vi "GetPositionWinCoords.vi"(8 "error in (no error)":errorcluster, 11 "reference in":refnum<class "SceneObject.lvclass">) -> (0 "error out":errorcluster, 2 "Position":T1, 3 "reference out":refnum<class "SceneObject.lvclass">)   [LabVIEW 2010, in "RenderBase.lvlib" / "SceneObject.lvclass"]
uses:
  SceneObject.lvclass
  <vilib>/Utility/miscctls.llb/LVPoint32TypeDef.ctl
  SceneRoot_class/SceneRoot.lvclass
  SceneRoot/GetSceneRoot.vi
  Position/GetPosition.vi
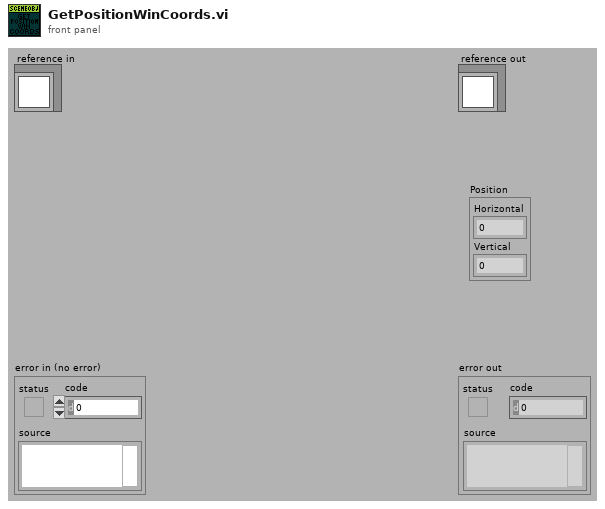
[diagram p1: front panel]
types:
  T1 = typedef "LVPoint32TypeDef.ctl" = cluster{"Horizontal":i32, "Vertical":i32}
  T2 = typedef "LV3DPointTypeDef.ctl" = cluster{"X":sgl, "Y":sgl, "Z":sgl}
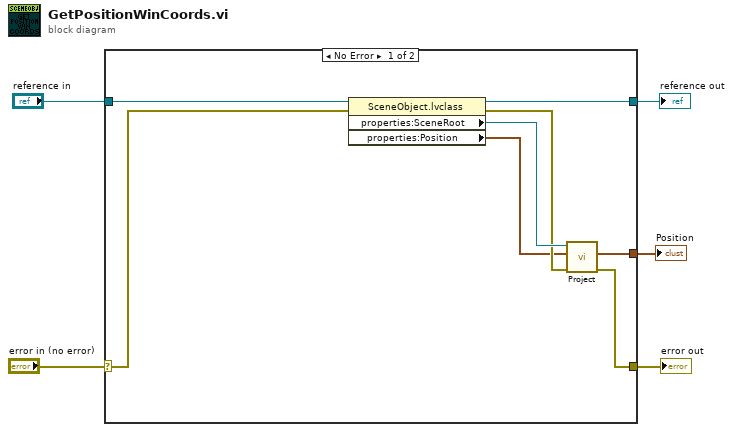
[diagram p0: block diagram]
diagram:
  n1 = case shown="No Error" "error in (no error)" {
    selector: "error in (no error)" -> [w11 w15]
    tunnel: [w7 w15] -> w4
    tunnel: [w9 w14] -> w2
    tunnel: "reference in" -> [w10 w14]
    tunnel: [w13 _] -> w1
    frame No Error {
      n2 = property class="SceneObject.lvclass"(reference=w10, error in=w11) -> (reference out=w9:refnum<class "SceneObject.lvclass">, error out=w8:errorcluster, "properties:SceneRoot"=w12:refnum<class "SceneRoot.lvclass">, "properties:Position"=w6:T2)
      n3 = call "Project.vi"("error in"=w8, "sceneCoords in"=w6, "class data in"=w12) -> ("error out"=w7:errorcluster, "winCoords out"=w13:T1)  [unwired: 6 in, 1 out]
    }
    frame Error {
    }
  }
  "error out" <- w4
  "reference out" <- w2
  "Position" <- w1
